vi "edit save.vi"(4 "Slide":refnum<vi>, 6 "appended path":path, 7 "filename":refnum<vi>, 8 "edit":bool, 9 "genneral info":string, 10 "tpdata":string[](array[string])) -> ()   [LabVIEW 2018]
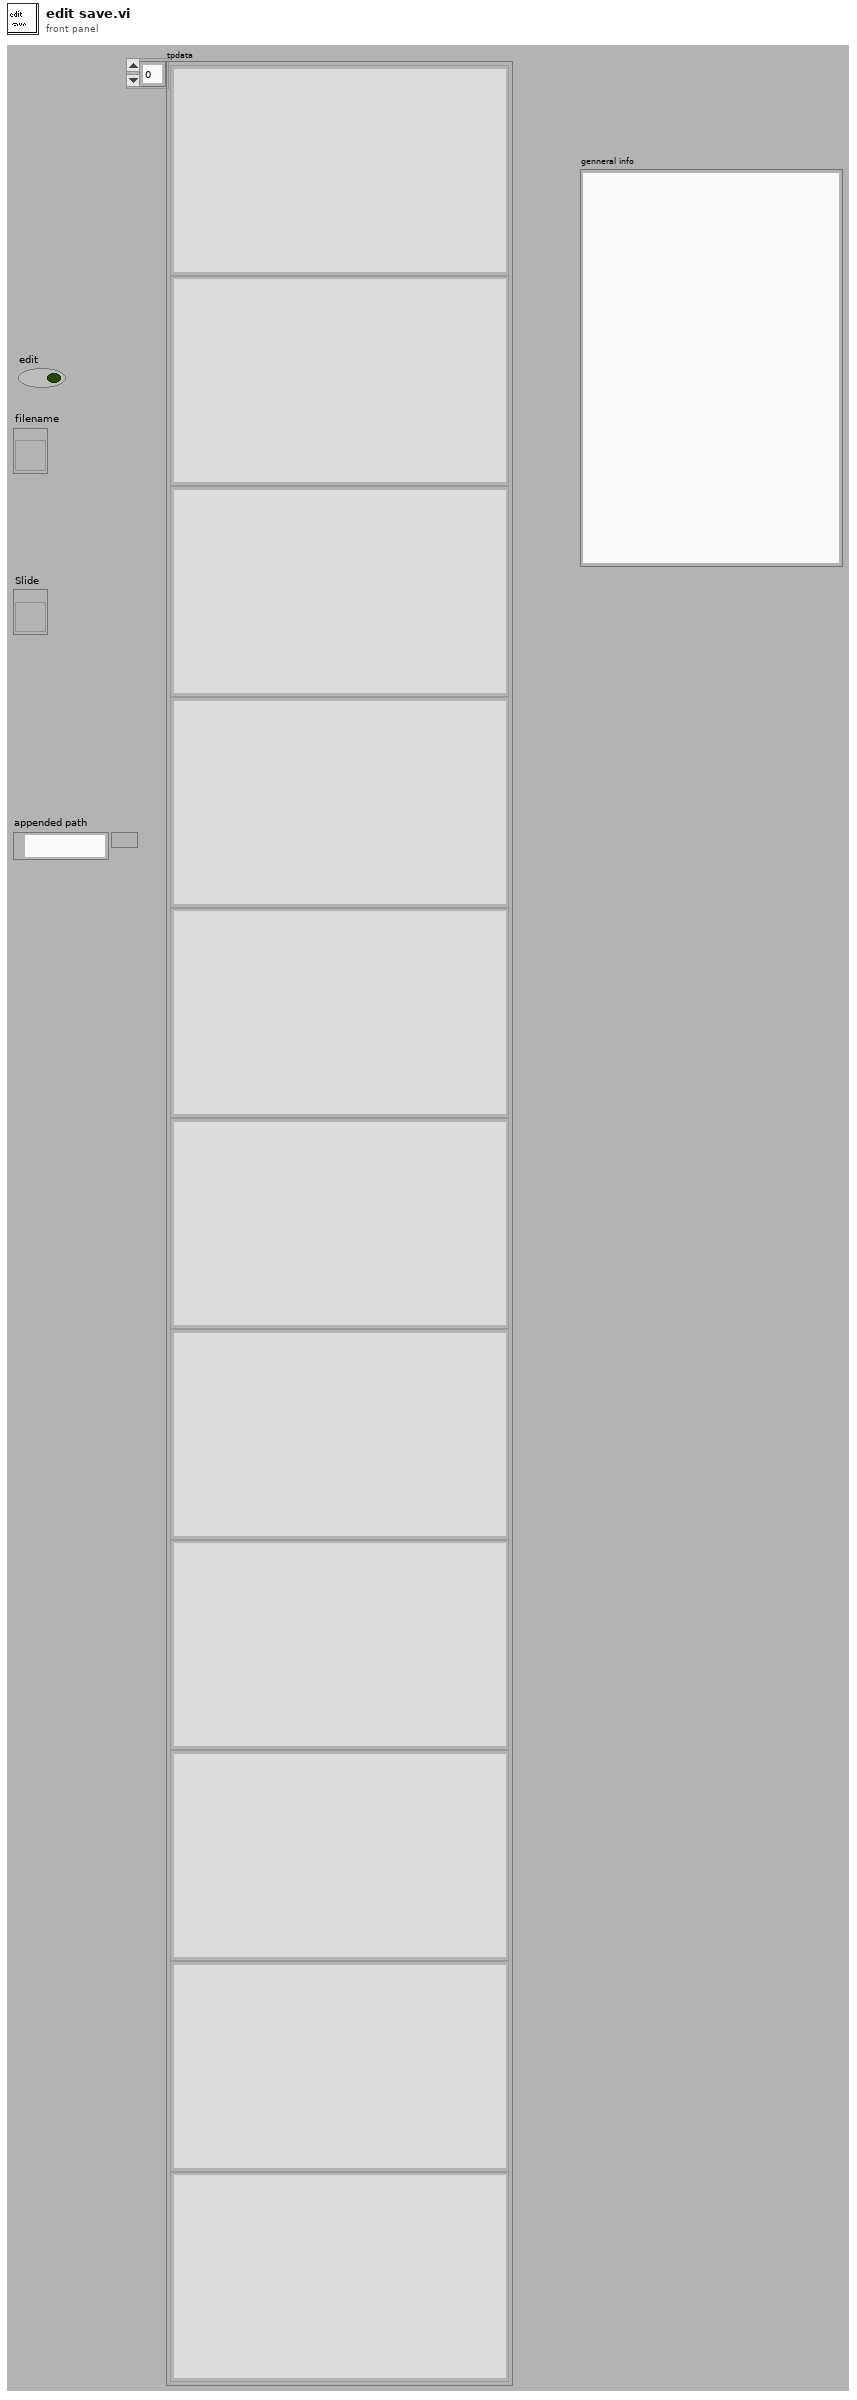
[diagram p1: front panel]
types:
  T1 = enum16{"open", "replace", "create", "open or create", "replace or create", "replace or create with confirmation"}
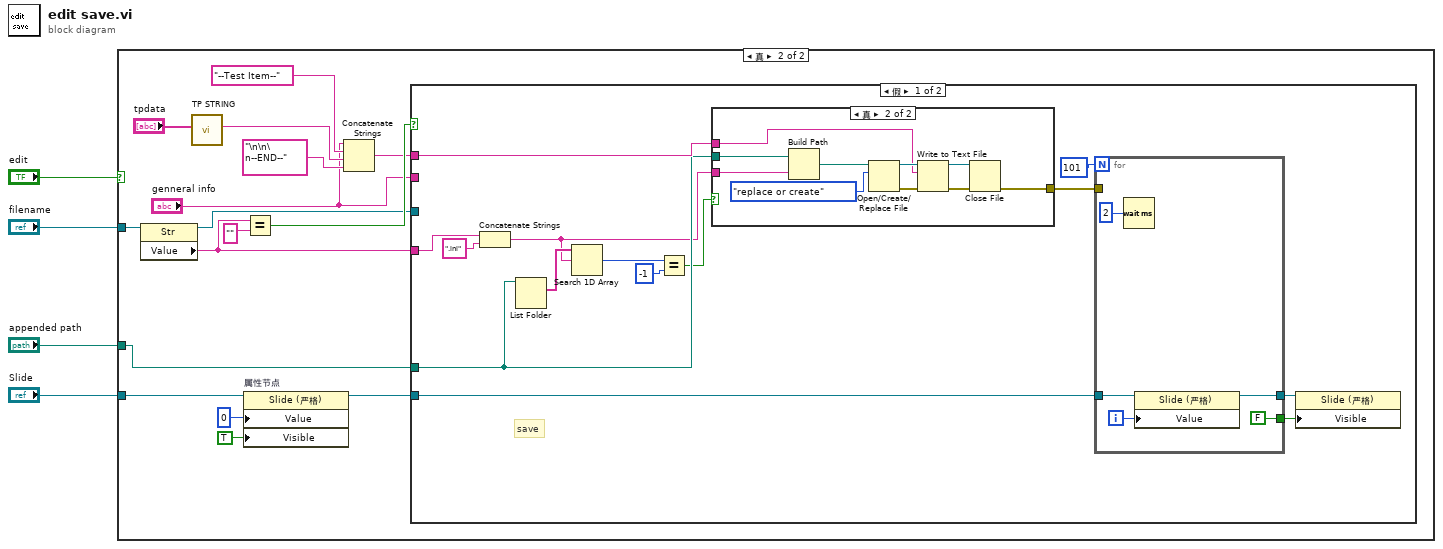
[diagram p0: block diagram]
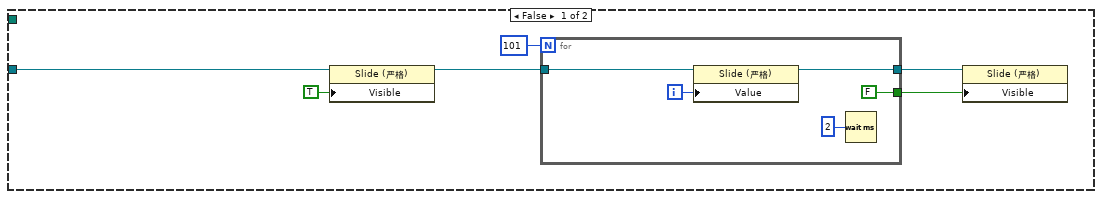
[diagram p2: hidden frame]
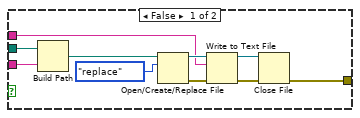
[diagram p3: hidden frame]
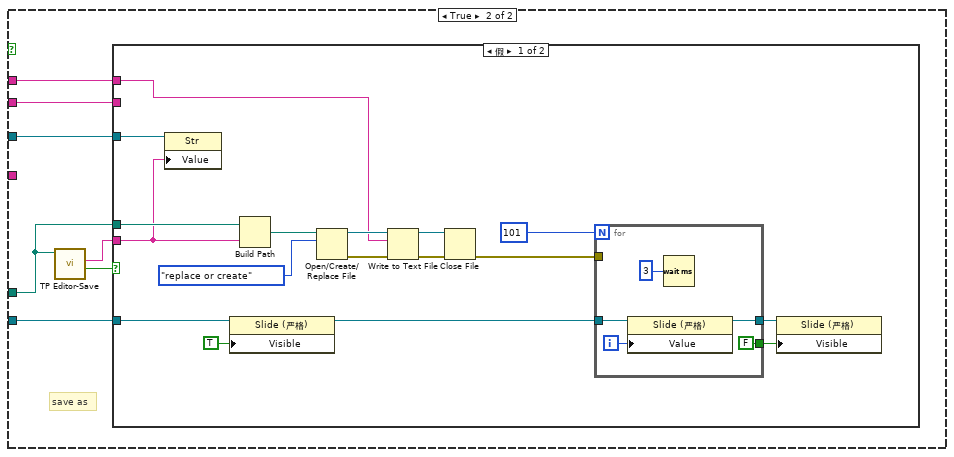
[diagram p4: hidden frame]
diagram:
  n1 = case shown="真" "edit" {
    tunnel: "appended path" -> [_ w17]
    tunnel: "filename" -> [_ w27]
    tunnel: "Slide" -> [w6 w21]
    frame False {
      n2 = property on="属性节点" class="Slide (严格)"(reference=w6, "Visible"=TRUE ("可见")) -> (reference out=w9:refnum<vi>)  [unwired: 1 in, 1 out]
      n3 = for {
        N: 101 -> [_]
        tunnel: [FALSE] -> w7
        tunnel: w9 -> [w12]
        tunnel: [w11] -> w8
        i -> [w15]
        n4 = property on="属性节点" class="Slide (严格)"(reference=w12, "Value"=w15) -> (reference out=w11:refnum<vi>)  [unwired: 1 in, 1 out]
        n5 = Wait (ms)(milliseconds to wait=u32 2) -> ()  [unwired: 1 out]
      }
      n6 = property on="属性节点" class="Slide (严格)"(reference=w8, "Visible"=w7) -> ()  [unwired: 1 in, 2 out]
    }
    frame True {
      n7 = property on="属性节点" class="Str"(reference=w27) -> (reference out=w22:refnum<vi>, "Value"=w29:string)  [unwired: 1 in, 1 out]
      n8 = call "TP STRING.vi"("tpdata"="tpdata") -> ("TP OUT"=w25:string)  [unwired: 1 in, 9 out]
      n9 = property on="属性节点" class="Slide (严格)"(reference=w21, "Value"=0, "Visible"=TRUE ("可见")) -> (reference out=w20:refnum<vi>)  [unwired: 1 in, 1 out]
      n10 = Equal?(x=w29, y="") -> (x = y?=w30:bool)
      n11 = Concatenate Strings("genneral info", "--Test Item--" ("字符串"), w25, "\n\n\n--END--") -> (w23:string)
      n12 = case shown="假" w30 {
        tunnel: w29 -> [w33 _]
        tunnel: w17 -> [w36 w76]
        tunnel: w20 -> [w41 w74]
        tunnel: w23 -> [w42 w73]
        tunnel: w22 -> [_ w72]
        tunnel: "genneral info" -> [_ w71]
        frame False {
          # "save"
          n13 = Concatenate Strings(w33, ".ini") -> (w32:string)
          n14 = List Folder(path=w36) -> (filenames=w39:string[])  [unwired: 1 in, 5 out]
          n15 = Search 1D Array(1D array=w39, element=w32) -> (index of element=w38:i32)  [unwired: 1 out]
          n16 = Equal?(x=w38, y=-1) -> (x = y?=w35:bool)
          n17 = case shown="真" w35 {
            tunnel: w36 -> [w47 w64]
            tunnel: w32 -> [w48 w56]
            tunnel: [w49 w60] -> w43
            tunnel: w42 -> [w46 w57]
            frame False {
              n18 = Build Path(base path=w47, name or relative path=w48) -> (appended path=w55:path)
              n19 = Open/Create/Replace File(file path (use dialog)=w55, operation (0:open)=T1."replace") -> (refnum out=w50:refnum<file>, error out=w51:errorcluster)  [unwired: 1 in, 4 out]
              n20 = Write to Text File(file (use dialog)=w50, text=w46, error in=w51) -> (refnum out=w53:refnum<file>, error out=w52:errorcluster)  [unwired: 2 out]
              n21 = Close File(refnum=w53, error in=w52) -> (error out=w49:errorcluster)  [unwired: 1 out]
            }
            frame True {
              n22 = Build Path(base path=w64, name or relative path=w56) -> (appended path=w65:path)
              n23 = Open/Create/Replace File(file path (use dialog)=w65, operation (0:open)=T1."replace or create") -> (refnum out=w58:refnum<file>, error out=w59:errorcluster)  [unwired: 1 in, 4 out]
              n24 = Write to Text File(file (use dialog)=w58, text=w57, error in=w59) -> (refnum out=w62:refnum<file>, error out=w61:errorcluster)  [unwired: 2 out]
              n25 = Close File(refnum=w62, error in=w61) -> (error out=w60:errorcluster)  [unwired: 1 out]
            }
          }
          n26 = for {
            N: 101 -> [_]
            tunnel: [FALSE] -> w44
            tunnel: w43 -> [_]
            tunnel: w41 -> [w67]
            tunnel: [w66] -> w40
            i -> [w70]
            n27 = Wait (ms)(milliseconds to wait=u32 2) -> ()  [unwired: 1 out]
            n28 = property on="属性节点" class="Slide (严格)"(reference=w67, "Value"=w70) -> (reference out=w66:refnum<vi>)  [unwired: 1 in, 1 out]
          }
          n29 = property on="属性节点" class="Slide (严格)"(reference=w40, "Visible"=w44) -> ()  [unwired: 1 in, 2 out]
        }
        frame True {
          # "save as"
          n30 = call "TP Editor-Save.vi"("path"=w76) -> ("Cancel"=w75:bool, "File Name 2"=w77:string)  [unwired: 1 in, 5 out]
          n31 = case shown="假" w75 {
            tunnel: w77 -> [w78 _]
            tunnel: w76 -> [w91 _]
            tunnel: w74 -> [w85 _]
            tunnel: w73 -> [w84 _]
            tunnel: w72 -> [w83 _]
            tunnel: w71 -> [_ _]
            frame False {
              n32 = property on="属性节点" class="Str"(reference=w83, "Value"=w78) -> ()  [unwired: 1 in, 2 out]
              n33 = property on="属性节点" class="Slide (严格)"(reference=w85, "Visible"=TRUE) -> (reference out=w82:refnum<vi>)  [unwired: 1 in, 1 out]
              n34 = Build Path(base path=w91, name or relative path=w78) -> (appended path=w86:path)
              n35 = Open/Create/Replace File(file path (use dialog)=w86, operation (0:open)=T1."replace or create") -> (refnum out=w94:refnum<file>, error out=w93:errorcluster)  [unwired: 1 in, 4 out]
              n36 = Write to Text File(file (use dialog)=w94, text=w84, error in=w93) -> (refnum out=w80:refnum<file>, error out=w79:errorcluster)  [unwired: 2 out]
              n37 = Close File(refnum=w80, error in=w79) -> (error out=w87:errorcluster)  [unwired: 1 out]
              n38 = for {
                N: 101 -> [_]
                tunnel: [FALSE] -> w89
                tunnel: w87 -> [_]
                tunnel: w82 -> [w96]
                tunnel: [w95] -> w81
                i -> [w99]
                n39 = property on="属性节点" class="Slide (严格)"(reference=w96, "Value"=w99) -> (reference out=w95:refnum<vi>)  [unwired: 1 in, 1 out]
                n40 = Wait (ms)(milliseconds to wait=u32 3) -> ()  [unwired: 1 out]
              }
              n41 = property on="属性节点" class="Slide (严格)"(reference=w81, "Visible"=w89) -> ()  [unwired: 1 in, 2 out]
            }
            frame True {
            }
          }
        }
      }
    }
  }
